vi "member_data_file_path_generate.vi"() -> (0 "appended path":path)   [LabVIEW 2014]
panel:
  out "name":string
  out "path":path
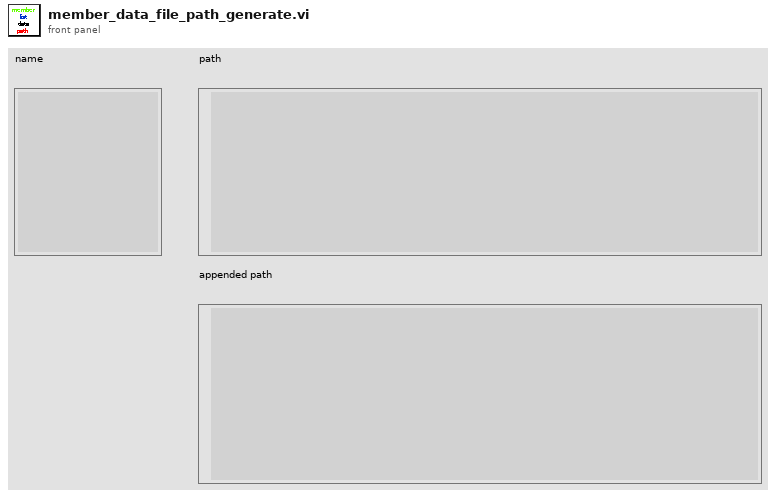
[diagram p1: front panel]
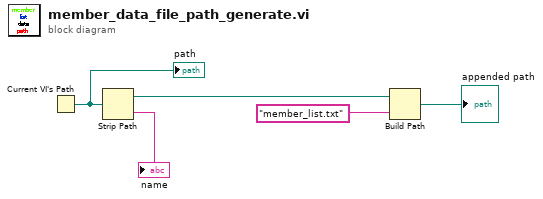
[diagram p0: block diagram]
diagram:
  n1 = Current VI's Path() -> (path=w5:path)
  "path" <- w5
  n2 = Strip Path(path=w5) -> (stripped path=w2:path, name=→"name":string)
  n3 = Build Path(base path=w2, name or relative path="member_list.txt") -> (appended path=→"appended path":path)
